vi "Flatten to 8-bit RGB.vi"(5 "AOI Overlay?":bool=TRUE, 6 "Pixel depth":u32, 7 "Black/White Levels":cluster{ext, ext}(slide)={1.0, 65535.0} scale=1.0..65535.0, 8 "error in":errorcluster, 9 "8 bit image buffer":T1, 10 "8 or 16 bit image in":T1, 11 "RGB Image buffer":T1) -> (0 "error out":errorcluster, 3 "RGB Image Out":T1)   [LabVIEW 2011]
doc: "Produces an intensity-scaled 8-bit RGB image (black and white) from either an 8- or 16-bit monochrome input."
uses:
  <vilib>/vision/Image Controls.llb/IMAQ Image.ctl
  <vilib>/vision/NI_Vision_Development_Module.lvlib
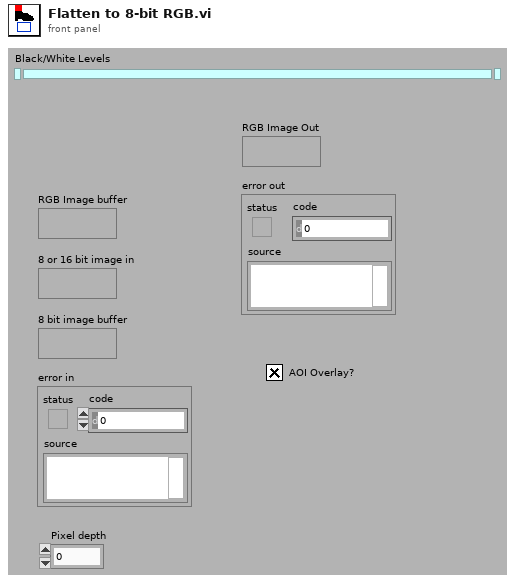
[diagram p1: front panel]
types:
  T1 = typedef "IMAQ Image.ctl" = refnum<image>
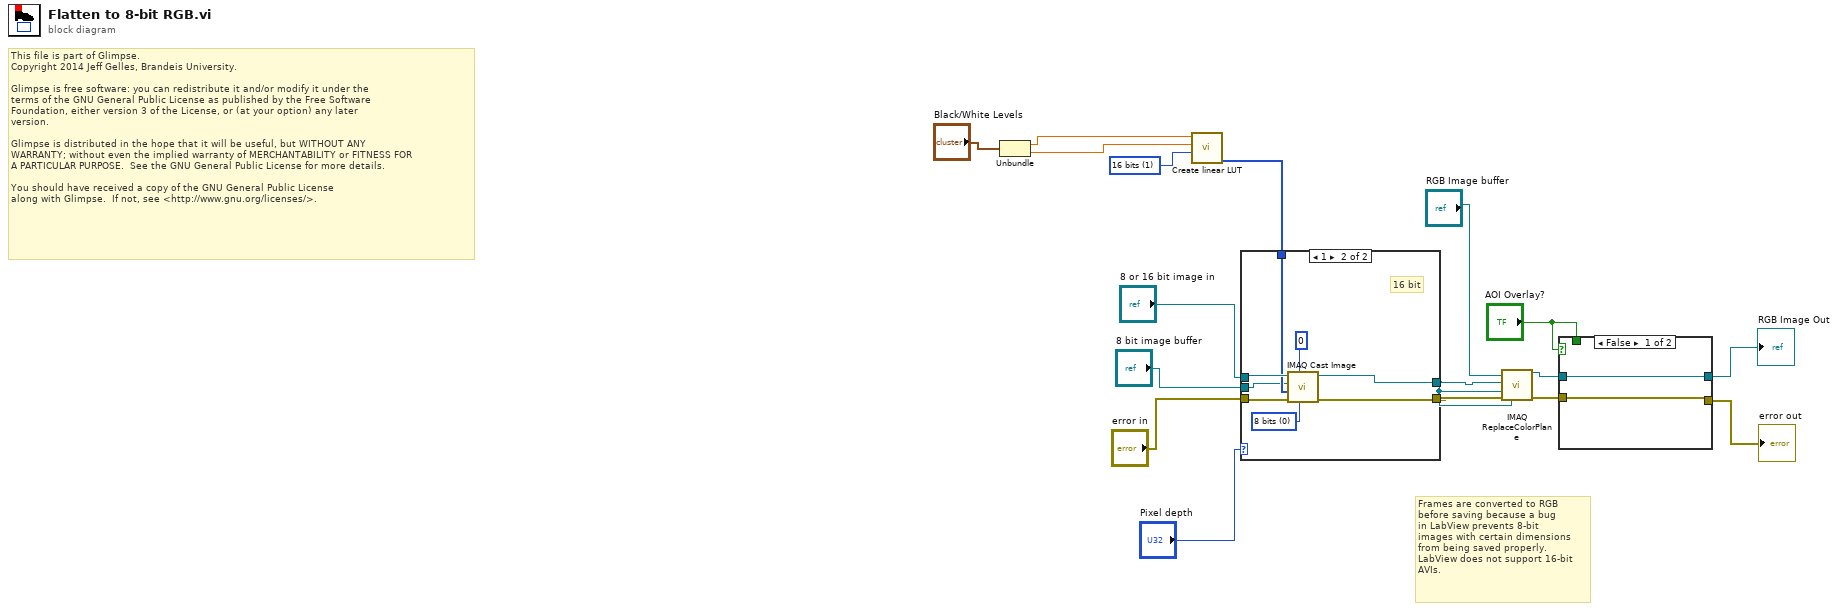
[diagram p0: block diagram]
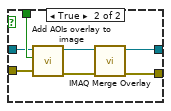
[diagram p2: hidden frame]
diagram:
  w10 = u32 1 items=["8 bits", "16 bits", "Float", "Complex", "RGB", "HSL"] ("Image Type")
  # "This file is part of Glimpse. \nCopyright 2014 Jeff Gelles, Brandeis University.    \n\nGlimpse is free software: you can redistribute it and/or modify it under the \nterms of the GNU General Public License as published by the Free Software \nFoundation, either version 3 of the License, or (at your option) any later \nversion.\n\nGlimpse is distributed in the hope that it will be useful, but WITHOUT ANY \nWARRANTY; without even the implied warranty of MERCHANTABILITY or FITNESS FOR \nA PARTICULAR PURPOSE.  See the GNU General Public License for more details.\n\nYou should have received a copy of the GNU General Public License\nalong with Glimpse.  If not, see <http://www.gnu.org/licenses/>."
  # "Frames are converted to RGB\nbefore saving because a bug\nin LabView prevents 8-bit \nimages with certain dimensions\nfrom being saved properly.\nLabView does not support 16-bit\nAVIs."
  n1 = Unbundle("Black/White Levels") -> (w8:ext, w9:ext)
  n2 = call "Create linear LUT.vi"("Input Image Type"=w10, "White Value"=w9, "Black Value"=w8) -> ("LUT (U8) Out"=w7:u8[])  [unwired: 1 in, 5 out]
  n3 = case shown="1" "Pixel depth" {
    tunnel: "8 or 16 bit image in" -> [w19 w26]
    tunnel: [w19 w20] -> w15
    tunnel: "error in" -> [w18 w27]
    tunnel: [w18 w21] -> w16
    tunnel: w7 -> [_ w25]
    tunnel: "8 bit image buffer" -> [_ w22]
    frame 0, Default {
      # "8-bit"
    }
    frame 1 {
      w23 = u32 0 items=["8 bits", "16 bits", "Float", "Complex", "RGB", "HSL"] ("Image Type")
      # "16 bit"
      n4 = call "IMAQ Cast Image"("Image Type"=w23, "# Shifts"=0, "error in (no error)"=w27, "Lookup Table"=w25, "Image Dst"=w22, "Image Src"=w26) -> ("error out"=w21:errorcluster, "Image Dst Out"=w20:T1)  [unwired: 4 out]
    }
  }
  n5 = call "IMAQ ReplaceColorPlane"("Image Dst"="RGB Image buffer", "Red or Hue Plane"=w15, "Green or Sat Plane"=w15, "error in (no error)"=w16, "Blue or Luma or Val or Inten Plane"=w15) -> ("Image Dst Out"=w3:T1, "error out"=w5:errorcluster)  [unwired: 2 in, 7 out]
  n6 = case shown="False" "AOI Overlay?" {
    tunnel: "AOI Overlay?" -> [_ w36]
    tunnel: w5 -> [w28 w35]
    tunnel: [w28 w31] -> w4
    tunnel: w3 -> [w29 w34]
    tunnel: [w29 w30] -> w2
    frame False {
    }
    frame True {
      n7 = call "Add AOIs overlay to image.vi"("error in (no error)"=w35, "Overlay on?"=w36, "Image Src"=w34) -> ("error out"=w33:errorcluster, "Image Dst"=w32:T1)  [unwired: 3 in, 4 out]
      n8 = call "IMAQ Merge Overlay"("error in (no error)"=w33, "Image Src"=w32) -> ("error out"=w31:errorcluster, "Image Dst Out"=w30:T1)  [unwired: 3 in, 5 out]
    }
  }
  "RGB Image Out" <- w2
  "error out" <- w4
